vi "Set_Report_Path.vi"(1 "测试板编号":i32, 2 "保存路径":path) -> (0 "创建生成路径":path)   [LabVIEW 2015]
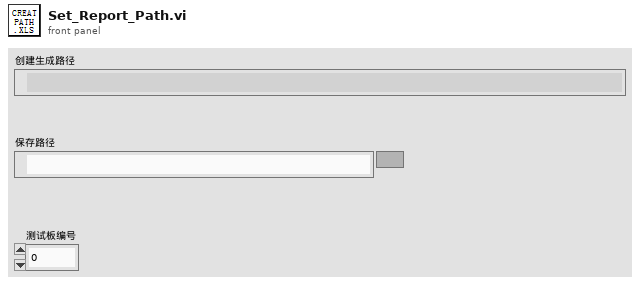
[diagram p1: front panel]
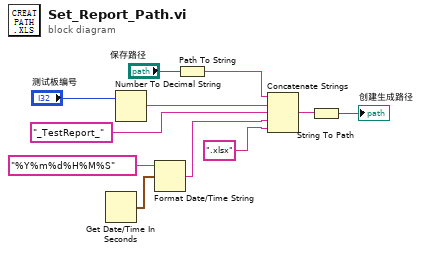
[diagram p0: block diagram]
diagram:
  n1 = Get Date/Time In Seconds() -> (seconds since 1Jan1904=w6:timestamp)
  n2 = Number To Decimal String(number="测试板编号") -> (decimal integer string=w8:string)  [unwired: 1 in]
  n3 = Format Date/Time String(time format string (%c)="%Y%m%d%H%M%S" ("时间格式字符串(%c)"), seconds (now)=w6) -> (date/time string=w4:string)  [unwired: 1 in]
  n4 = Path To String(path="保存路径") -> (string=w10:string)
  n5 = Concatenate Strings(w10, w8, "_TestReport_", w4, ".xlsx") -> (w2:string)
  n6 = String To Path(string=w2) -> (path=→"创建生成路径":path)
